vi "Material-Line3-TestMain.vi"(8 "error in (no error)":errorcluster, 11 "Material-RunTest in":refnum<class "Material-RunTest.lvclass">) -> (0 "error out":errorcluster, 3 "Material-RunTest out":refnum<class "Material-RunTest.lvclass">)   [LabVIEW 2013, in "Material-RunTest.lvclass"]
uses:
  Material-RunTest.lvclass
  Material-RunTest.lvclass/Material-RunTest.ctl
  Motion Control/Motion-ControlAll.lvclass
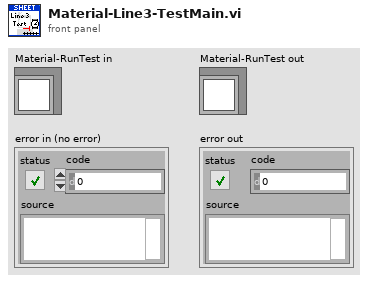
[diagram p1: front panel]
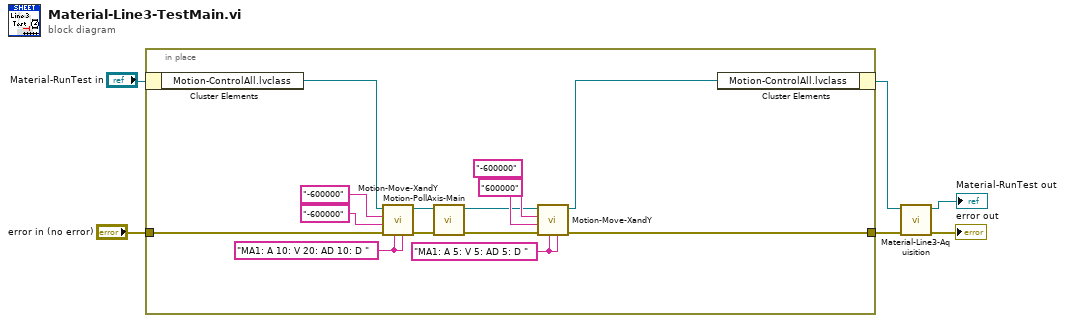
[diagram p0: block diagram]
diagram:
  n1 = in-place {
    in-place-border: "error in (no error)" -> [w20]
    in-place-border: [w7] -> w4
    w8 = "MA1: A 10: V 20: AD 10: D " ("X Drive Acc/Speed/Velocity")
    w9 = "MA1: A 5: V 5: AD 5: D " ("concatenated string")
    n2 = in-place-cluster #1("Material-RunTest in") -> ("Motion-ControlAll.lvclass"=w19:refnum<class "Motion-ControlAll.lvclass">)
    n3 = call "Motion-Move-XandY.vi"("Y Drive Acc/Speed/Velocity"=w8, "X Drive Acc/Speed/Velocity"=w8, "error in (no error)"=w20, "X Coordinates"="-600000", "Y Coordinates"="-600000", "Motion-ControlAll in"=w19) -> ("error out"=w17:errorcluster, "Motion-ControlAll out"=w18:refnum<class "Motion-ControlAll.lvclass">)  [unwired: 4 in]
    n4 = call "Motion-PollAxis-Main.vi"("error in (no error)"=w17, "Motion-ControlAll in"=w18) -> ("error out"=w12:errorcluster, "Motion-ControlAll out"=w11:refnum<class "Motion-ControlAll.lvclass">)  [unwired: 8 in]
    n5 = call "Motion-Move-XandY.vi"("Y Drive Acc/Speed/Velocity"=w9, "X Drive Acc/Speed/Velocity"=w9, "error in (no error)"=w12, "X Coordinates"="600000", "Y Coordinates"="-600000", "Motion-ControlAll in"=w11) -> ("error out"=w7:errorcluster, "Motion-ControlAll out"=w10:refnum<class "Motion-ControlAll.lvclass">)  [unwired: 4 in]
    n6 = in-place-cluster #1("Motion-ControlAll.lvclass"=w10) -> (w3:refnum<class "Material-RunTest.lvclass">)
  }
  n7 = call "Material-Line3-Aquisition.vi"("error in (no error)"=w4, "Material-RunTest in"=w3) -> ("error out"=→"error out":errorcluster, "Material-RunTest out"=→"Material-RunTest out":refnum<class "Material-RunTest.lvclass">)  [unwired: 8 in]
